vi "stop.vi"(8 "error in (no error)":errorcluster, 10 "Stop abruptly? (T)":bool=TRUE, 11 "Picomotor in":refnum<class "Newport Model 8742.lvclass">) -> (0 "error out":errorcluster, 3 "Picomotor out":refnum<class "Newport Model 8742.lvclass">)   [LabVIEW 2020, in "Newport Model 8742.lvclass"]
uses:
  Newport Model 8742.lvclass
  Newport Model 8742.lvclass/Newport Model 8742.ctl
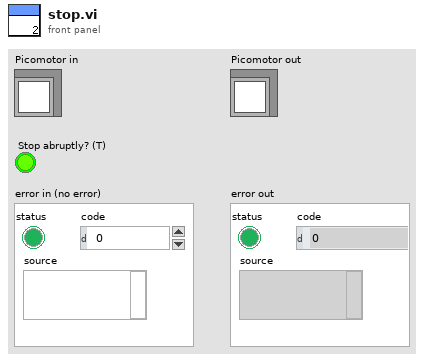
[diagram p1: front panel]
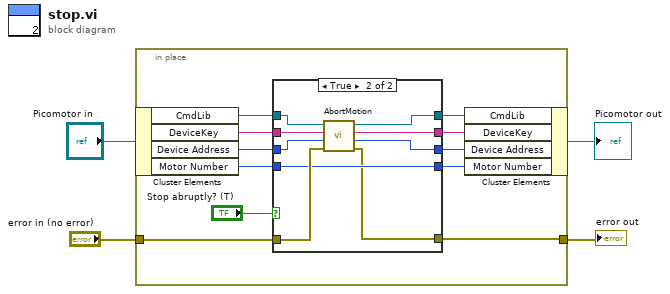
[diagram p0: block diagram]
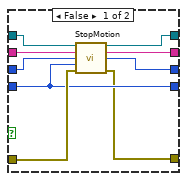
[diagram p2: hidden frame]
diagram:
  n1 = in-place {
    in-place-border: "error in (no error)" -> [w10]
    in-place-border: [w5] -> w1
    n2 = in-place-cluster #1("Picomotor in") -> ("CmdLib"=w14:refnum<k24>, "DeviceKey"=w13:string, "Device Address"=w12:i32, "Motor Number"=w11:i32)
    n3 = case shown="True" "Stop abruptly? (T)" {
      tunnel: w14 -> [w18 w30]
      tunnel: w13 -> [w21 w31]
      tunnel: w12 -> [w22 w29]
      tunnel: w11 -> [w23 w32]
      tunnel: w10 -> [w24 w33]
      tunnel: [w23 w32] -> w9
      tunnel: [w19 w28] -> w8
      tunnel: [w20 w27] -> w7
      tunnel: [w17 w26] -> w6
      tunnel: [w16 w25] -> w5
      frame False {
        n4 = call <instrlib>:"StopMotion.vi"("CmdLib In"=w18, "DeviceKey In"=w21, "Device Address In"=w22, "Motor"=w23, "error in (no error)"=w24) -> ("CmdLib Out"=w17:refnum<k24>, "DeviceKey Out"=w20:string, "Device Address Out"=w19:i32, "error out"=w16:errorcluster)  [unwired: 7 in]
      }
      frame True {
        n5 = call <instrlib>:"AbortMotion.vi"("error in (no error)"=w33, "Device Address In"=w29, "DeviceKey In"=w31, "CmdLib In"=w30) -> ("error out"=w25:errorcluster, "Device Address Out"=w28:i32, "DeviceKey Out"=w27:string, "CmdLib Out"=w26:refnum<k24>)
      }
    }
    n6 = in-place-cluster #1("CmdLib"=w6, "DeviceKey"=w7, "Device Address"=w8, "Motor Number"=w9) -> (→"Picomotor out":refnum<class "Newport Model 8742.lvclass">)
  }
  "error out" <- w1
